vi "find channel tag indicies.vi"(10 "channels":refnum<class "TBM channel.lvclass">[](array[class]), 11 "data allocations":T2) -> (0 "Output Indicies":T1, 1 "Result Indicies":T1, 2 "Parameter Indicies":T1, 3 "Input Indicies":T1)   [LabVIEW 2013]
uses:
  <vilib>/NI/Tag Bus Module Framework/channel/data tables.ctl
  <vilib>/NI/Tag Bus/dictionary/data dictionary.lvclass
  <vilib>/NI/Tag Bus/dictionary table pair.ctl
  <vilib>/NI/Tag Bus/table/data table.ctl
  <vilib>/NI/Tag Bus Module Framework/channel/TBM channel.lvclass
  Cluster to Tag Bus Scripts/Channel Run Time Mapping Info.ctl
  <vilib>/NI/Tag Bus Module Framework/channel/TBM channel.lvclass/TBM channel.ctl
  <vilib>/NI/Tag Bus/tag/tag descriptor.lvclass/tag descriptor.ctl
  <vilib>/NI/Tag Bus/tag/tag descriptor.lvclass
  <vilib>/NI/Tag Bus/table/data table.lvlib
  <vilib>/NI/Tag Bus/tag bus.lvlib
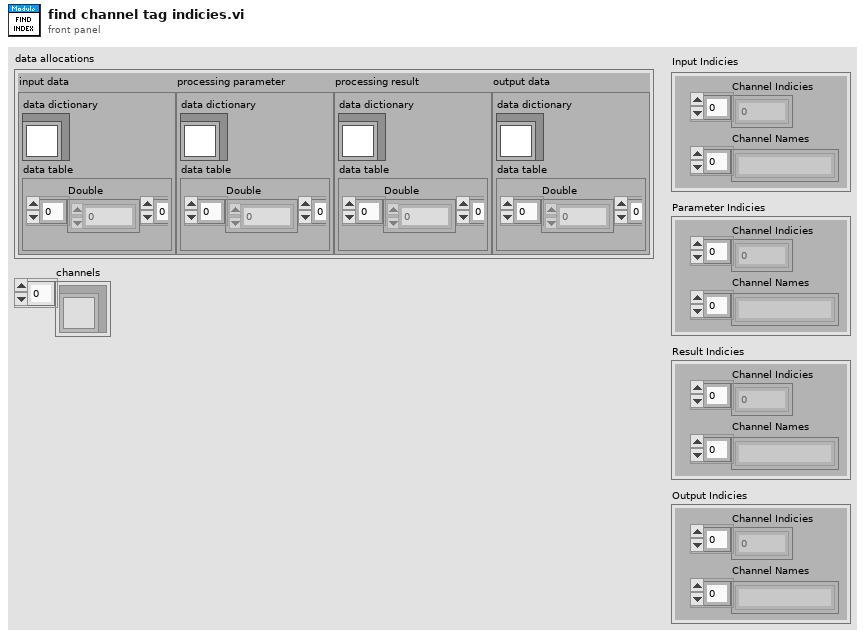
[diagram p1: front panel]
types:
  T1 = typedef "Channel Run Time Mapping Info.ctl" = cluster{"Channel Indicies":i32[], "Channel Names":string[]}
  T2 = typedef "TBM channel.lvclass/data tables.ctl" = cluster{"input data":T3, "processing parameter":T3, "processing result":T3, "output data":T3}
  T3 = typedef "tag bus.lvlib/dictionary table pair.ctl" = cluster{"data dictionary":refnum<class "data dictionary.lvclass">, "data table":T4}
  T4 = typedef "tag bus.lvlib/data table.lvlib/data table.ctl" = cluster{"Double":dbl[], "Single":sgl[], "I64":i64[], "I32":i32[], "I16":i16[], "I8":i8[], "U64":u64[], "U32":u32[], "U16":u16[], "U8":u8[], "Boolean":bool[], "String":string[], "Array of Double":cluster{"DBL Array":dbl[]}[], "Array of Single":cluster{"SGL Array":sgl[]}[], "Array of I64":cluster{"I64 Array":i64[]}[], "Array of I32":cluster{"I32 Array":i32[]}[], "Array of I16":cluster{"I16 Array":i16[]}[], "Array of I8":cluster{"I8 Array":i8[]}[], "Array of U64":cluster{"U64 Array":u64[]}[], "Array of U32":cluster{"U32 Array":u32[]}[], "Array of U16":cluster{"U16 Array":u16[]}[], "Array of U8":cluster{"U8 Array":u8[]}[], "Array of Boolean":cluster{"Boolean Array":bool[]}[], "Array of String":cluster{"String Array":string[]}[]}
  T5 = typedef "TBM channel.lvclass/channel classification.ctl" = enum16{"input data", "output data", "processing parameter", "processing result"}
  T6 = typedef "tag bus.lvlib/tag descriptor.lvclass/Data Type.ctl" = enum16{"Double", "Single", "I64", "I32", "I16", "I8", "U64", "U32", "U16", "U8", "Boolean", "String", "Array of Double", "Array of Single", "Array of I64", "Array of I32", "Array of I16", "Array of I8", "Array of U64", "Array of U32", "Array of U16", "Array of U8", "Array of Boolean", "Array of String"}
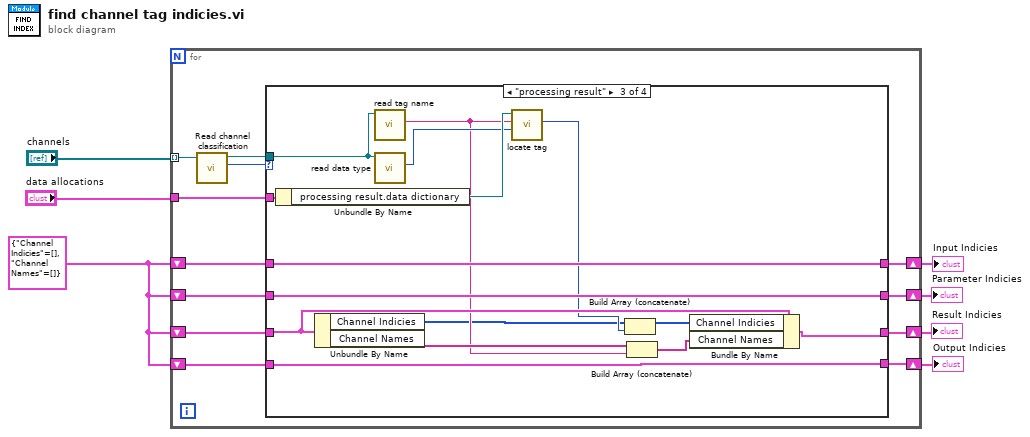
[diagram p0: block diagram]
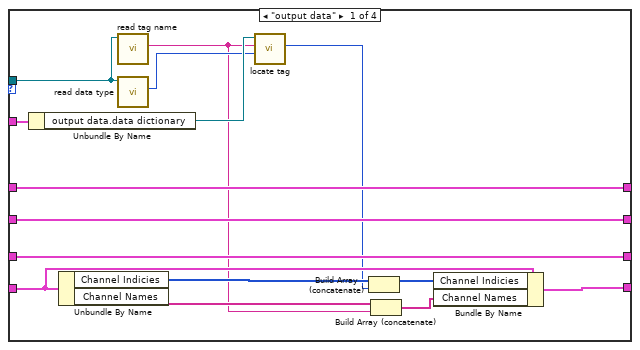
[diagram p2: hidden frame]
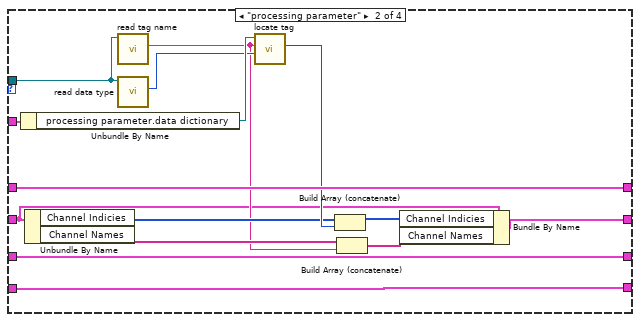
[diagram p3: hidden frame]
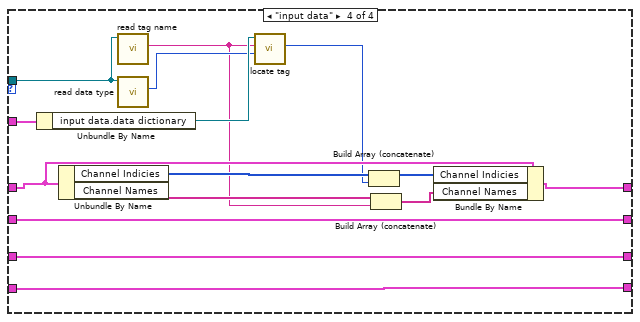
[diagram p4: hidden frame]
diagram:
  w2 = T1 {"Channel Indicies"=[], "Channel Names"=[]} ("Input Indicies")
  n1 = for {
    tunnel: "channels" -> [w19] mode=indexing
    tunnel: "data allocations" -> [w17]
    shift-right: [w11] -> w1
    shift-left: w2 -> [w15]
    shift-right: [w10] -> w5
    shift-left: w2 -> [w14]
    shift-right: [w8] -> w4
    shift-left: w2 -> [w13]
    shift-right: [w9] -> w3
    shift-left: w2 -> [w12]
    n2 = call <vilib>:"Read channel classification.vi"("channel in"=w19) -> ("channel classification"=w18:T5, "channel out"=w16:refnum<class "TBM channel.lvclass">)  [unwired: 8 in, 1 out]
    n3 = case shown="\"processing result\"" w18 {
      tunnel: w17 -> [w34 w49 w64 w79]
      tunnel: w16 -> [w32 w47 w62 w77]
      tunnel: w15 -> [w30 w45 w60 w67]
      tunnel: w14 -> [w29 w38 w58 w74]
      tunnel: w13 -> [w28 w44 w55 w73]
      tunnel: w12 -> [w23 w42 w59 w75]
      tunnel: [w30 w45 w60 w68] -> w11
      tunnel: [w29 w35 w58 w74] -> w10
      tunnel: [w22 w42 w59 w75] -> w9
      tunnel: [w28 w44 w52 w73] -> w8
      frame "output data" {
        n4 = Unbundle By Name(w34) -> ("output data.data dictionary"=w33:refnum<class "data dictionary.lvclass">)
        n5 = Unbundle By Name(w23) -> ("Channel Indicies"=w25:i32[], "Channel Names"=w27:string[])
        n6 = call <vilib>:"read tag name.vi"("system tag in"=w32) -> ("name"=w21:string)  [unwired: 8 in, 2 out]
        n7 = call <vilib>:"read data type.vi"("system tag in"=w32) -> ("data type"=w31:T6)  [unwired: 8 in, 2 out]
        n8 = call <vilib>:"locate tag.vi"("data type"=w31, "name"=w21, "data dictionary in"=w33) -> ("index"=w20:i32)  [unwired: 6 in, 2 out]
        n9 = Build Array (concatenate)(w25, w20) -> (w26:i32[])
        n10 = Build Array (concatenate)(w27, w21) -> (w24:string[])
        n11 = Bundle By Name(cluster=w23, "Channel Indicies"=w26, "Channel Names"=w24) -> (w22:T1)
      }
      frame "processing parameter" {
        n12 = Unbundle By Name(w49) -> ("processing parameter.data dictionary"=w48:refnum<class "data dictionary.lvclass">)
        n13 = Unbundle By Name(w38) -> ("Channel Indicies"=w41:i32[], "Channel Names"=w40:string[])
        n14 = call <vilib>:"read tag name.vi"("system tag in"=w47) -> ("name"=w39:string)  [unwired: 8 in, 2 out]
        n15 = call <vilib>:"read data type.vi"("system tag in"=w47) -> ("data type"=w46:T6)  [unwired: 8 in, 2 out]
        n16 = call <vilib>:"locate tag.vi"("data type"=w46, "name"=w39, "data dictionary in"=w48) -> ("index"=w43:i32)  [unwired: 6 in, 2 out]
        n17 = Build Array (concatenate)(w41, w43) -> (w37:i32[])
        n18 = Build Array (concatenate)(w40, w39) -> (w36:string[])
        n19 = Bundle By Name(cluster=w38, "Channel Indicies"=w37, "Channel Names"=w36) -> (w35:T1)
      }
      frame "processing result" {
        n20 = Unbundle By Name(w64) -> ("processing result.data dictionary"=w63:refnum<class "data dictionary.lvclass">)
        n21 = Unbundle By Name(w55) -> ("Channel Indicies"=w51:i32[], "Channel Names"=w57:string[])
        n22 = call <vilib>:"read tag name.vi"("system tag in"=w62) -> ("name"=w53:string)  [unwired: 8 in, 2 out]
        n23 = call <vilib>:"read data type.vi"("system tag in"=w62) -> ("data type"=w61:T6)  [unwired: 8 in, 2 out]
        n24 = call <vilib>:"locate tag.vi"("data type"=w61, "name"=w53, "data dictionary in"=w63) -> ("index"=w54:i32)  [unwired: 6 in, 2 out]
        n25 = Build Array (concatenate)(w51, w54) -> (w56:i32[])
        n26 = Build Array (concatenate)(w57, w53) -> (w50:string[])
        n27 = Bundle By Name(cluster=w55, "Channel Indicies"=w56, "Channel Names"=w50) -> (w52:T1)
      }
      frame "input data" {
        n28 = Unbundle By Name(w79) -> ("input data.data dictionary"=w78:refnum<class "data dictionary.lvclass">)
        n29 = Unbundle By Name(w67) -> ("Channel Indicies"=w70:i32[], "Channel Names"=w72:string[])
        n30 = call <vilib>:"read tag name.vi"("system tag in"=w77) -> ("name"=w66:string)  [unwired: 8 in, 2 out]
        n31 = call <vilib>:"read data type.vi"("system tag in"=w77) -> ("data type"=w76:T6)  [unwired: 8 in, 2 out]
        n32 = call <vilib>:"locate tag.vi"("data type"=w76, "name"=w66, "data dictionary in"=w78) -> ("index"=w65:i32)  [unwired: 6 in, 2 out]
        n33 = Build Array (concatenate)(w70, w65) -> (w71:i32[])
        n34 = Build Array (concatenate)(w72, w66) -> (w69:string[])
        n35 = Bundle By Name(cluster=w67, "Channel Indicies"=w71, "Channel Names"=w69) -> (w68:T1)
      }
    }
  }
  "Parameter Indicies" <- w5
  "Result Indicies" <- w4
  "Output Indicies" <- w3
  "Input Indicies" <- w1
